vi "grabber stage control panel.vi"() -> ()   [LabVIEW 2010]
uses:
  location3D.ctl
  ASI-stage/stage properties.ctl
panel:
  in  "Wave Specs":T1={"XAmp"=0.0, "YAmp"=0.0, "Zamp"=0.0, "T (sec)"=10.0, "Wave Type"=enum."Sine"}
  in  "output wave?":bool
  in  "large deviation override":T2={"x (um)"=600.0, "y (um)"=800.0, "Poverride"=1.2}
  out "file write error":bool
  out "file access error":bool
  out "error out":errorcluster
  in  "set pcros (um)":cluster{"X":dbl, "Y":dbl, "Z":dbl}={"X"=0.02, "Y"=0.02, "Z"=0.02}
  in  "deadband (um)":dbl=0.1
  out "tracker location":T3
  out "z move (um)":dbl
  out "y move (um)":dbl
  out "x move (um)":dbl
  in  "HALT":bool
  out "out of range":bool
  out "limits":T4
  out "stage initialized":bool
  in  "move stage":bool
  in  "target":cluster{"X ":dbl, "Y ":dbl, "Z ":dbl} {"Z" format="%#.4f"; "Y" format="%#.4f"; "X" format="%#.4f"}
  out "location":cluster{"X ":dbl, "Y ":dbl, "Z ":dbl} {"Z" format="%#.4f"; "Y" format="%#.4f"; "X" format="%#.4f"}
  in  "z range (um)":dbl=200.0
  in  "xy range (um)":dbl=10000.0
  in  "update period (ms)":u32=25
  in  "Baud rate":u32=115200
  in  "stage com port":refnum<visa-resource-name>="COM9"
  in  "set stage boundaries":bool
  in  "close stage":bool
  in  "open stage":bool
  in  "stop":bool
  out "stage location":cluster{"X out":dbl, "Y out":dbl, "Z out":dbl}(graph)
  in  "Z gains":T5={"proportional gain (Kc)"=0.35, "integral time (Ti, sec)"=15.0, "derivative time (Td, sec)"=0.0} {"derivative time (Td, sec)" format="%.3f"; "integral time (Ti, sec)" format="%.3f"; "proportional gain (Kc)" format="%.3f"}
  in  "XY gains":T5={"proportional gain (Kc)"=0.35, "integral time (Ti, sec)"=15.0, "derivative time (Td, sec)"=0.0} {"derivative time (Td, sec)" format="%.3f"; "integral time (Ti, sec)" format="%.3f"; "proportional gain (Kc)" format="%.3f"}
  in  "feedback polarity":T6={"x polarity"=TRUE, "y polarity"=FALSE, "z polarity"=FALSE}
  in  "engage stage feedback":bool
  out "tracking":bool
  in  "focalPositionQueue":refnum<queue>
  # "correct (tuned) parameters = 0.35, 15, 0"
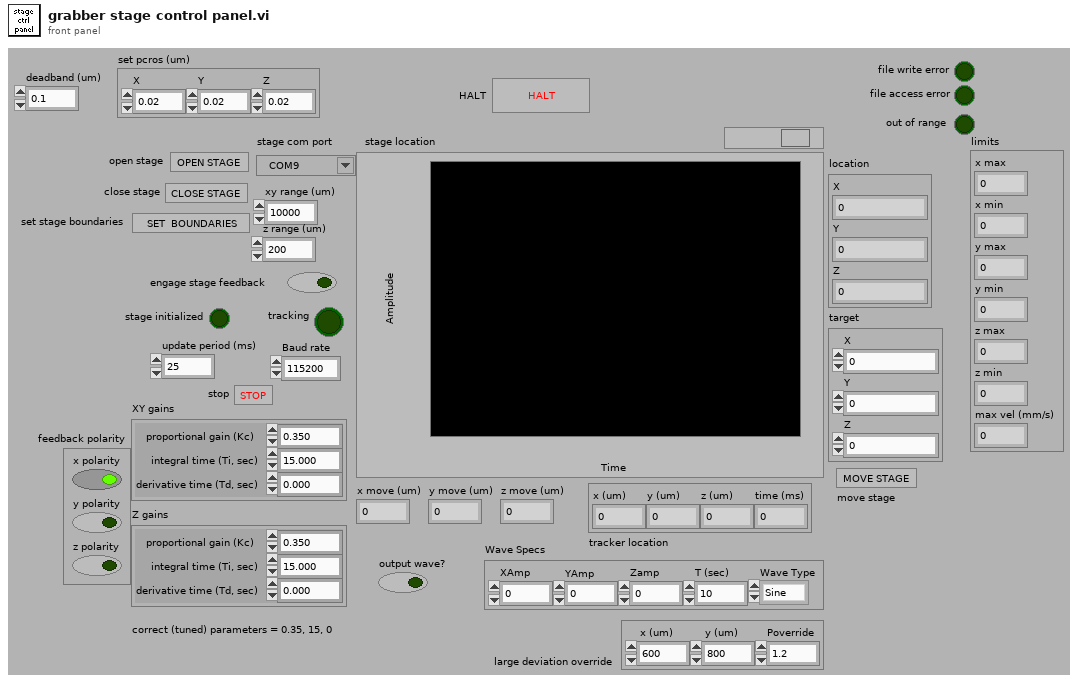
[diagram p1: front panel]
types:
  T1 = cluster{"XAmp":dbl, "YAmp":dbl, "Zamp":dbl, "T (sec)":dbl, "Wave Type":enum16{"Sine", "Triange"}}
  T2 = cluster{"x (um)":dbl, "y (um)":dbl, "Poverride":dbl}
  T3 = cluster{"x (um)":dbl, "y (um)":dbl, "z (um)":dbl, "time (ms)":i64}
  T4 = cluster{"x max":dbl, "x min":dbl, "y max":dbl, "y min":dbl, "z max":dbl, "z min":dbl, "max vel (mm/s)":dbl}
  T5 = cluster{"proportional gain (Kc)":dbl, "integral time (Ti, sec)":dbl, "derivative time (Td, sec)":dbl}
  T6 = cluster{"x polarity":bool, "y polarity":bool, "z polarity":bool}
  T7 = typedef "stage properties.ctl" = cluster{"VISA resource name":refnum<visa-resource-name>, "limits":cluster{"x max":dbl, "x min":dbl, "y max":dbl, "y min":dbl, "z max":dbl, "z min":dbl, "max vel (mm/s)":dbl}, "initialized":bool, "PCROS":cluster{"X":dbl, "Y":dbl, "Z":dbl}}
  T8 = typedef "location3D.ctl" = cluster{"x (um)":dbl, "y (um)":dbl, "z (um)":dbl, "time (ms)":i64}
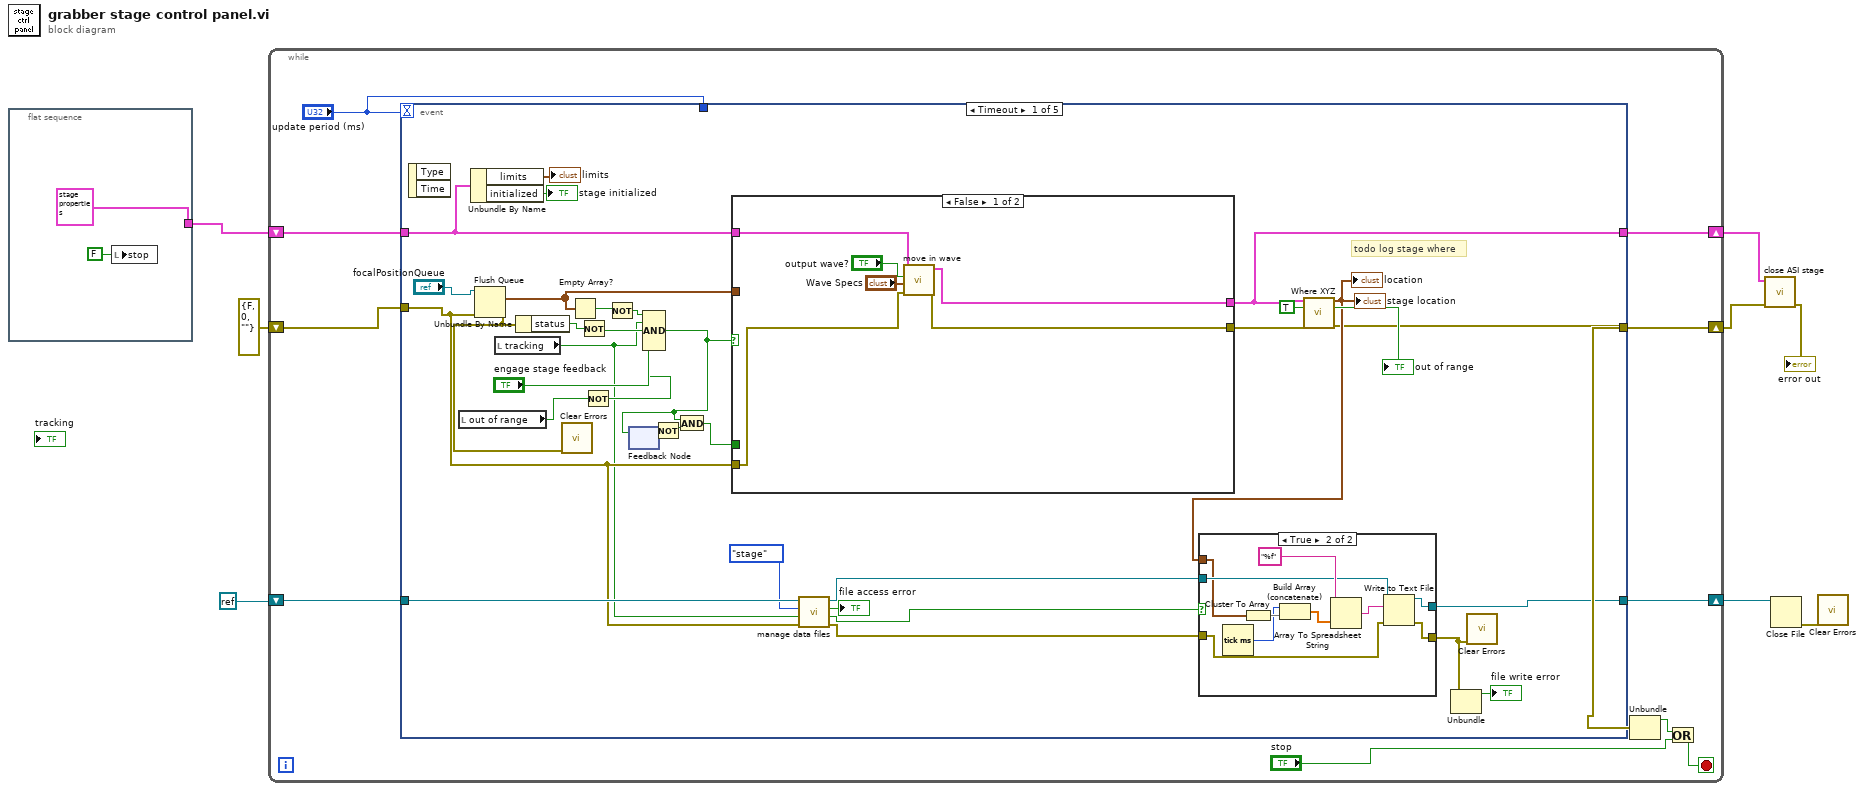
[diagram p0: block diagram]
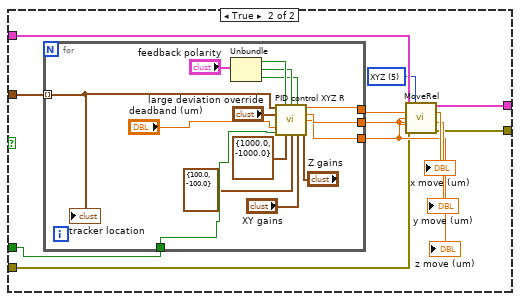
[diagram p3: hidden frame]
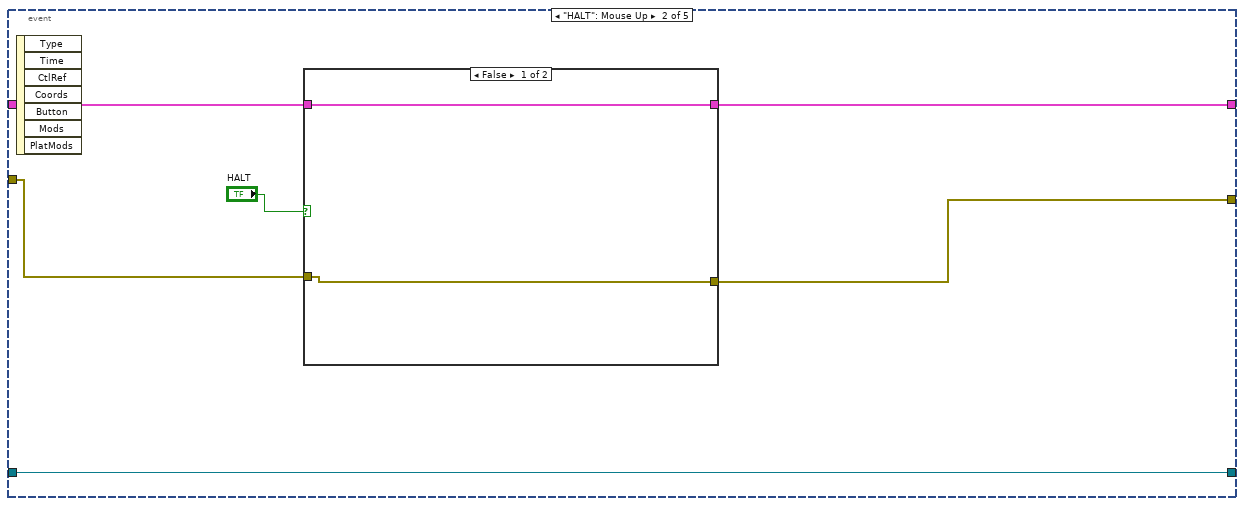
[diagram p4: hidden frame]
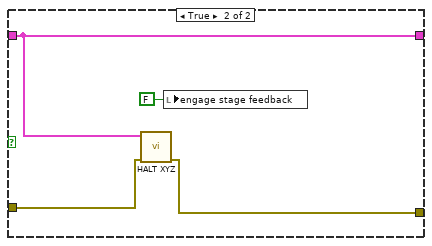
[diagram p5: hidden frame]
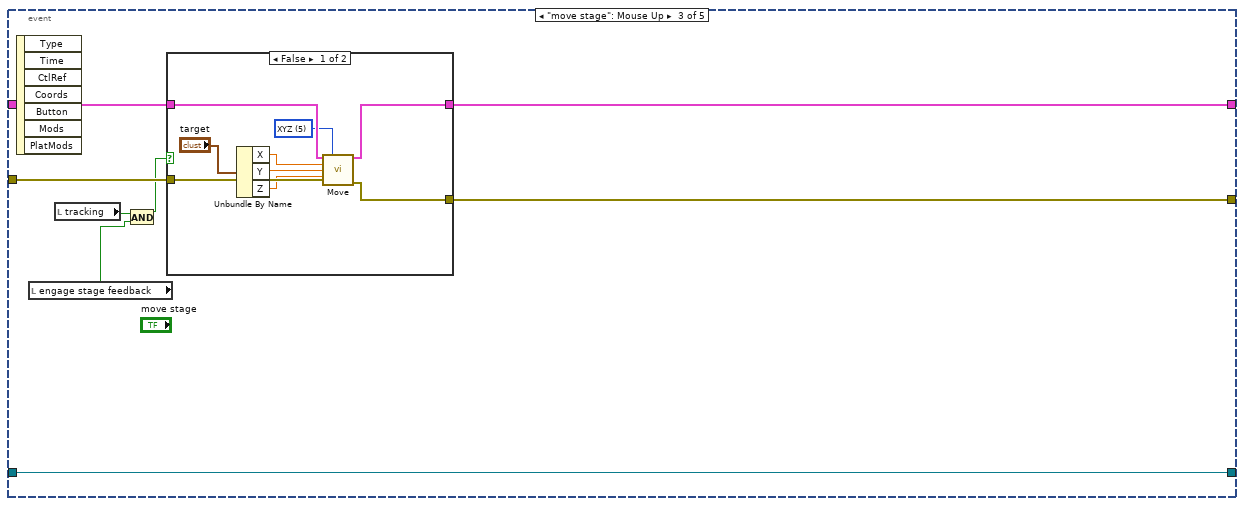
[diagram p6: hidden frame]
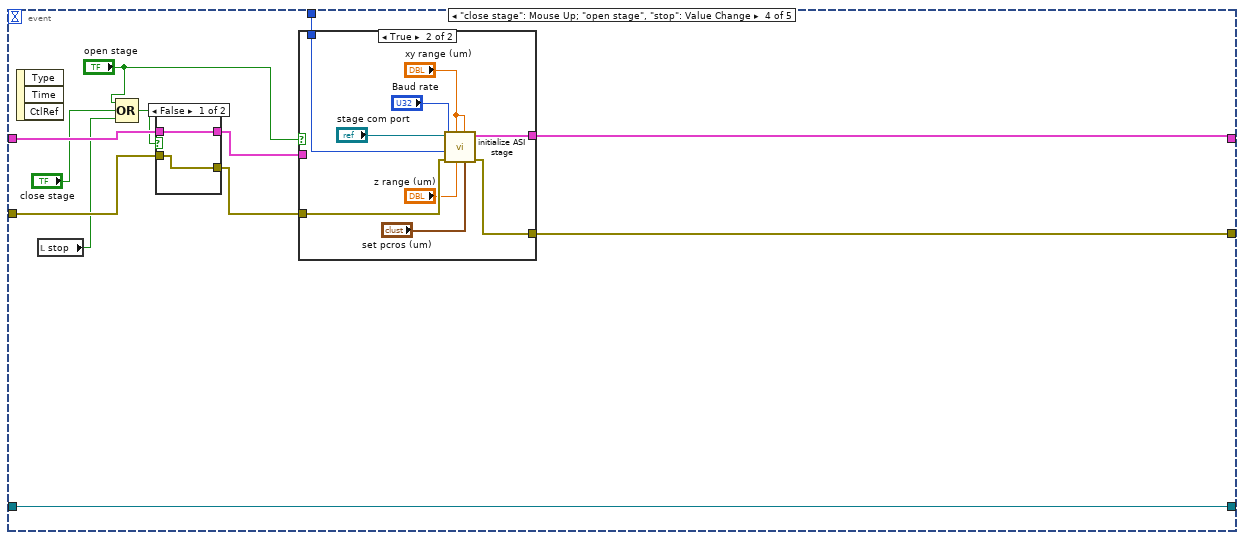
[diagram p8: hidden frame]
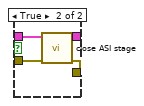
[diagram p9: hidden frame]
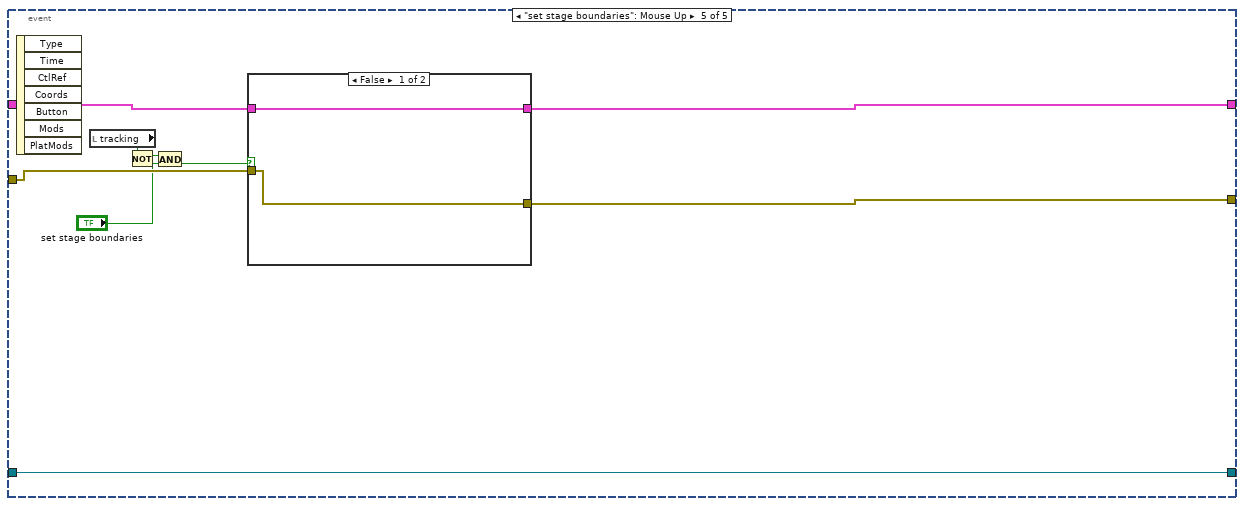
[diagram p11: hidden frame]
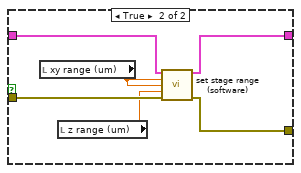
[diagram p12: hidden frame]
diagram:
  n1 = flat-sequence {
    tunnel: [T7 {"VISA resource name"="", "limits"={"x max"=0.0, "x min"=0.0, "y max"=0.0, "y min"=0.0, "z max"=0.0, "z min"=0.0, "max vel (mm/s)"=0.0}, "initialized"=FALSE, "PCROS"={"X"=0.0, "Y"=0.0, "Z"=0.0}} ("ASI stage")] -> w7
    frame #0 {
      n2 = local write "stop"(FALSE ("stop")) -> ()
    }
  }
  n3 = while {
    shift-right: [w17] -> w5
    shift-left: w7 -> [w19]
    shift-right: [w16] -> w6
    shift-left: errorcluster {"status"=FALSE, "code"=0, "source"=""} ("error out") -> [w18]
    shift-right: [w11] -> w2
    shift-left: refnum<k0> refnum -> [w10]
    stop <- w14 stop-if-true
    n4 = event shown="[0] Timeout" {
      selector: _ -> [_ _ _ _ _]
      dyn-events: _ -> [_ _ _ _ _]
      timeout: "update period (ms)" -> [_ _ _ _ _]
      tunnel: w19 -> [w43 w101 w115 w137 w165]
      tunnel: [w22 w99 w113 w139 w163] -> w16
      tunnel: w18 -> [w31 w100 w116 w136 w164]
      tunnel: [w44 w98 w114 w138 w162] -> w17
      tunnel: "update period (ms)" -> [_ _ _ w129 _]
      tunnel: [w23 w97 w109 w128 w157] -> w11
      tunnel: w10 -> [w32 w97 w109 w128 w157]
      event Timeout {
        # "todo log stage where"
        n5 = event-data() -> ()  [unwired: 1 in, 2 out]
        n6 = local read "out of range"() -> (w38:bool)
        n7 = Unbundle By Name(w43) -> ("limits"=→"limits":T4, "initialized"=→"stage initialized":bool)
        n8 = Flush Queue(queue="focalPositionQueue", error in (no error)=w31) -> (remaining elements=w50:T8[], error out=w33:errorcluster)  [unwired: 1 out]
        n9 = local read "tracking"() -> (w29:bool)
        n10 = Unbundle By Name(w33) -> ("status"=w35:bool)
        n11 = call <vilib>:"Clear Errors.vi"("error in (no error)"=w33) -> ()  [unwired: 6 in, 1 out]
        n12 = Empty Array?(array=w50) -> (empty?=w52:bool)
        n13 = Not(x=w35) -> (.not. x?=w34:bool)
        n14 = Not(x=w38) -> (.not. x?=w37:bool)
        n15 = Not(x=w52) -> (.not. x?=w51:bool)
        n16 = feedback #1() -> (w49:bool)  [unwired: 1 in]
        n17 = Compound Arithmetic op=AND(w51, w29, w34, "engage stage feedback", w37) -> (w36:bool)
        n18 = feedback-in #1(w36) -> ()
        n19 = Not(x=w49) -> (.not. x?=w48:bool)
        n20 = And(x=w36, y=w48) -> (x .and. y?=w47:bool)
        n21 = case shown="False" w36 {
          tunnel: w50 -> [_ w81]
          tunnel: w47 -> [_ w80]
          tunnel: w43 -> [w71 w79]
          tunnel: w31 -> [w69 w75]
          tunnel: [w68 w73] -> w46
          tunnel: [w70 w72] -> w44
          frame False {
            n22 = call "move in wave.vi"("error in (no error)"=w69, "Wave Specs"="Wave Specs", "output wave?"="output wave?", "ASI stage"=w71) -> ("error out"=w68:errorcluster, "ASI stage out"=w70:T7)  [unwired: 6 in]
          }
          frame True {
            w74 = u16 5 items=["No axis", "X", "Y", "Z", "XY", "XYZ"] ("Axis configuration")
            n23 = for {
              tunnel: w81 -> [w84] mode=indexing
              tunnel: w80 -> [w96]
              tunnel: [w87] -> w78
              tunnel: [w86] -> w77
              tunnel: [w85] -> w76
              n24 = Unbundle("feedback polarity") -> ("x polarity"=w94:bool, "y polarity"=w93:bool, "z polarity"=w92:bool)
              n25 = call "PID control XYZ R.vi"("location"=w84, "x polarity"=w94, "y polarity"=w93, "z polarity"=w92, "large deviation override"="large deviation override", "deadband (um)"="deadband (um)", "reinitialize? (F)"=w96, "XY pos range (um)"=cluster{"output high":dbl, "output low":dbl} {"output high"=1000.0, "output low"=-1000.0}, "z position range (um)"=cluster{"output high":dbl, "output low":dbl} {"output high"=100.0, "output low"=-100.0}, "XY gains"="XY gains", "Z gains"="Z gains") -> ("x move (um)"=w87:dbl, "y move (um)"=w86:dbl, "z move (um)"=w85:dbl)  [unwired: 2 in]
              "tracker location" <- w84
            }
            "x move (um)" <- w78
            "y move (um)" <- w77
            "z move (um)" <- w76
            n26 = call "MoveRel.vi"("ASI stage"=w79, "Axis configuration"=w74, "x"=w78, "y"=w77, "z"=w76, "error in (no error)"=w75) -> ("ASI stage out"=w72:T7, "error out"=w73:errorcluster)  [unwired: 8 in]
          }
        }
        n27 = call "manage data files.vi"("error in"=w31, "tracking"=w29, "recording type"=enum16{"tracking", "stage"}."stage", "refnum in"=w32) -> ("error out"=w26:errorcluster, "file open for writing"=w27:bool, "file access error"=→"file access error":bool, "refnum out"=w24:refnum<file>)  [unwired: 4 in]
        n28 = call "Where XYZ.vi"("ASI stage"=w44, "stop if out of range"=TRUE, "error in (no error)"=w46) -> ("location"=w25:cluster{"X out":dbl, "Y out":dbl, "Z out":dbl}, "out of range"=→"out of range":bool, "error out"=w22:errorcluster)  [unwired: 10 in]
        "stage location" <- w25
        "location" <- w25
        n29 = case shown="True" w27 {
          tunnel: w26 -> [w54 w61]
          tunnel: w25 -> [_ w59]
          tunnel: w24 -> [w55 w63]
          tunnel: [w55 w62] -> w23
          tunnel: [w54 w60] -> w21
          frame False {
          }
          frame True {
            n30 = Tick Count (ms)() -> (millisecond timer value=w57:u32)
            n31 = Cluster To Array(cluster=w59) -> (array=w58:dbl[])
            n32 = Build Array (concatenate)(w57, w58) -> (w56:dbl[])
            n33 = Array To Spreadsheet String(array=w56, 3:"%f" ("format (%.3f)")) -> (spreadsheet string=w64:string)  [unwired: 1 in]
            n34 = Write to Text File(file (use dialog)=w63, text=w64, error in=w61) -> (refnum out=w62:refnum<file>, error out=w60:errorcluster)  [unwired: 1 in, 1 out]
          }
        }
        n35 = Unbundle(w21) -> ("status"=→"file write error":bool)  [unwired: 2 out]
        n36 = call <vilib>:"Clear Errors.vi"("error in (no error)"=w21) -> ()  [unwired: 6 in, 1 out]
      }
      event "HALT": Mouse Up {
        n37 = event-data() -> ()  [unwired: 1 in, 7 out]
        n38 = case shown="False" "HALT" {
          tunnel: w101 -> [w104 w106]
          tunnel: w100 -> [w103 w108]
          tunnel: [w103 w107] -> w99
          tunnel: [w104 w106] -> w98
          frame False {
          }
          frame True {
            n39 = call "HALT XYZ.vi"("error in (no error)"=w108, "ASI stage"=w106) -> ("error out"=w107:errorcluster)  [unwired: 9 in]
            n40 = local write "engage stage feedback"(FALSE ("engage stage feedback")) -> ()
          }
        }
      }
      event "move stage": Mouse Up {
        n41 = event-data() -> ()  [unwired: 1 in, 7 out]
        n42 = local read "engage stage feedback"() -> (w110:bool)
        n43 = local read "tracking"() -> (w112:bool)
        n44 = And(x=w112, y=w110) -> (x .and. y?=w111:bool)
        n45 = case shown="False" w111 {
          tunnel: w116 -> [w125 w126]
          tunnel: w115 -> [w124 w127]
          tunnel: [w123 w127] -> w114
          tunnel: [w122 w126] -> w113
          frame False {
            w121 = u16 5 items=["No axis", "X", "Y", "Z", "XY", "XYZ"] ("Axis configuration")
            n46 = Unbundle By Name("target") -> ("X"=w119:dbl, "Y"=w118:dbl, "Z"=w117:dbl)
            n47 = call "Move.vi"("ASI stage"=w124, "Axis configuration"=w121, "x"=w119, "y"=w118, "z"=w117, "error in (no error)"=w125) -> ("ASI stage out"=w123:T7, "error out"=w122:errorcluster)  [unwired: 8 in]
          }
          frame True {
          }
        }
      }
      event "close stage": Mouse Up; "open stage", "stop": Value Change {
        n48 = event-data() -> ()  [unwired: 1 in, 3 out]
        n49 = local read "stop"() -> (w131:bool)
        n50 = Compound Arithmetic op=OR("open stage", "close stage", w131) -> (w130:bool)
        n51 = case shown="False" w130 {
          tunnel: w137 -> [w141 w145]
          tunnel: w136 -> [w140 w144]
          tunnel: [w140 w143] -> w135
          tunnel: [w141 w142] -> w134
          frame False {
          }
          frame True {
            n52 = call "close ASI stage.vi"("error in (no error)"=w144, "ASI stage"=w145) -> ("error out"=w143:errorcluster, "ASI stage out"=w142:T7)  [unwired: 8 in]
          }
        }
        n53 = case shown="True" "open stage" {
          tunnel: w135 -> [w146 w154]
          tunnel: [w146 w151] -> w139
          tunnel: [w147 w150] -> w138
          tunnel: w134 -> [w147 _]
          tunnel: w129 -> [_ w148]
          frame False {
          }
          frame True {
            n54 = call "initialize ASI stage.vi"("set pcros (um)"="set pcros (um)", "y range"="xy range (um)", "z range"="z range (um)", "x range"="xy range (um)", "error in (no error)"=w154, "timeout"=w148, "Baud rate"="Baud rate", "VISA resource name"="stage com port") -> ("error out"=w151:errorcluster, "ASI stage"=w150:T7)  [unwired: 2 in]
          }
        }
      }
      event "set stage boundaries": Mouse Up {
        n55 = event-data() -> ()  [unwired: 1 in, 7 out]
        n56 = local read "tracking"() -> (w161:bool)
        n57 = Not(x=w161) -> (.not. x?=w159:bool)
        n58 = And(x="set stage boundaries", y=w159) -> (x .and. y?=w160:bool)
        n59 = case shown="False" w160 {
          tunnel: w165 -> [w167 w173]
          tunnel: w164 -> [w166 w172]
          tunnel: [w166 w171] -> w163
          tunnel: [w167 w170] -> w162
          frame False {
          }
          frame True {
            n60 = local read "xy range (um)"() -> (w169:dbl)
            n61 = local read "z range (um)"() -> (w168:dbl)
            n62 = call "set stage range (software).vi"("ASI stage"=w173, "x range"=w169, "y range"=w169, "z range"=w168, "error in (no error)"=w172) -> ("ASI stage out"=w170:T7, "error out"=w171:errorcluster)  [unwired: 9 in]
          }
        }
      }
    }
    n63 = Unbundle(w16) -> ("status"=w15:bool)  [unwired: 2 out]
    n64 = Or(x=w15, y="stop") -> (x .or. y?=w14:bool)
  }
  "error out" <- w6
  n65 = call "close ASI stage.vi"("error in (no error)"=w6, "ASI stage"=w5) -> ()  [unwired: 8 in, 2 out]
  n66 = Close File(refnum=w2) -> (error out=w1:errorcluster)  [unwired: 1 in, 1 out]
  n67 = call <vilib>:"Clear Errors.vi"("error in (no error)"=w1) -> ()  [unwired: 6 in, 1 out]
